vi "Create UI Pointers.vi"(8 "error in (no error)":errorcluster) -> (0 "error out":errorcluster, 3 "UI Pointers":T1)   [LabVIEW 2017]
uses:
  User Interface Pointers.ctl
  <vilib>/NI/Memory Manager/Classes/Pointer/Pointer.lvclass
  <vilib>/NI/Memory Manager/Classes/Pointer/Pointer.lvclass/Pointer.ctl
  <vilib>/NI/Memory Manager/Classes/Pointer/Write U32.vi
  <vilib>/NI/Memory Manager/Classes/Pointer/Write Bool.vi
  <vilib>/NI/Memory Manager/Classes/Pointer/Set Address.vi
  <vilib>/NI/Memory Manager/Classes/Pointer/Set Size.vi
  <vilib>/NI/Memory Manager/Classes/Pointer/Set Internal.vi
  <vilib>/NI/Memory Manager/Classes/Pointer/Clear.vi
  <vilib>/NI/Memory Manager/Classes/Pointer/Write (No Check).vi
  <vilib>/NI/Memory Manager/Classes/Pointer/Write (No Check) U32.vi
  <vilib>/NI/Memory Manager/Classes/Pointer/Check Move.vi
  <vilib>/NI/Memory Manager/Classes/Pointer/Write (No Check) Bool.vi
  <vilib>/NI/Memory Manager/Classes/Pointer/Check Null Pointer.vi
  <vilib>/NI/Memory Manager/Classes/Pointer/Clear (No Check).vi
  <vilib>/NI/Memory Manager/Classes/Pointer/Check Length.vi
  <vilib>/NI/Memory Manager/Classes/Pointer/Get Address.vi
  <vilib>/NI/Memory Manager/Classes/Pointer/Check Count.vi
  <vilib>/NI/Memory Manager/Classes/Pointer/Check Bounds (Power of 2).vi
  <vilib>/NI/Memory Manager/Classes/Pointer/Errors.vi
  <vilib>/NI/Memory Manager/Classes/Pointer/Null Pointer.vi
  <vilib>/NI/Memory Manager/Classes/Pointer/Is Null.vi
  <vilib>/NI/Memory Manager/Classes/Pointer/Get Size.vi
  <vilib>/NI/Memory Manager/Classes/Pointer/Check Bounds (Pointer).vi
  <vilib>/NI/Memory Manager/Classes/Pointer/Out of Bounds.vi
  <vilib>/NI/Memory Manager/Classes/Pointer/Check Bounds.vi
  <vilib>/NI/Memory Manager/Classes/Pointer/Create Error.vi
  <vilib>/NI/Memory Manager/Classes/Pointer/Write Pointer Size to Error.vi
  <vilib>/NI/Memory Manager/Classes/Pointer/Check Bounds (Buffer).vi
  <vilib>/NI/Memory Manager/Constants/Constants.vi
  <vilib>/NI/Memory Manager/Constants/Library Name.vi
  <vilib>/NI/Memory Manager/Classes/Pointer/Pointer Error Info.vi
  <vilib>/NI/Memory Manager/Constants/Pointer Class Name.vi
  <vilib>/NI/Memory Manager/Classes/Pointer/Buffer Underflow.vi
  <vilib>/NI/Memory Manager/VIs/New Error Cluster.vi
  <vilib>/NI/Memory Manager/VIs/New Error Cluster (512B).vi
  <vilib>/NI/Memory Manager/VIs/Set Error Status.vi
  <vilib>/NI/Memory Manager/VIs/Set Error Code.vi
  <vilib>/NI/Memory Manager/VIs/Set Error Source.vi
  <vilib>/NI/Memory Manager/VIs/Write String to Source.vi
  <vilib>/NI/Memory Manager/VIs/Write Numeric to Source.vi
  <vilib>/NI/Memory Manager/VIs/Write Numeric Scalar to Source (Base10 U64).vi
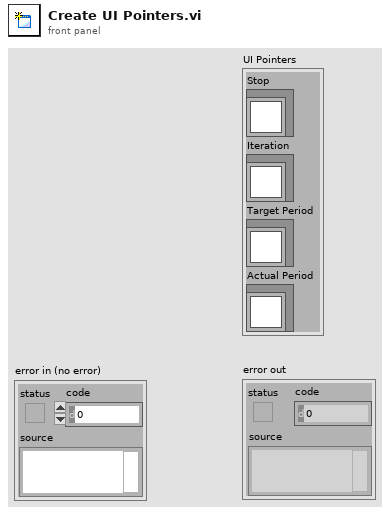
[diagram p1: front panel]
types:
  T1 = typedef "User Interface Pointers.ctl" = cluster{"Stop":refnum<class "Pointer.lvclass">, "Iteration":refnum<class "Pointer.lvclass">, "Target Period":refnum<class "Pointer.lvclass">, "Actual Period":refnum<class "Pointer.lvclass">}
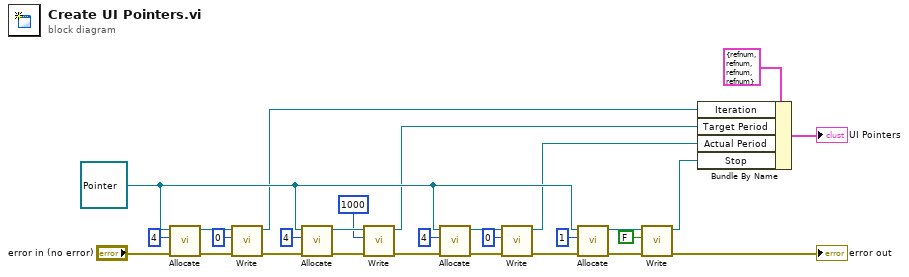
[diagram p0: block diagram]
diagram:
  w13 = refnum<class "Pointer.lvclass"> refnum ("Pointer in")
  n1 = call <vilib>:"Allocate.vi"("error in (no error)"="error in (no error)", "size"=u64 4, "Pointer type"=w13) -> ("error out"=w18:errorcluster, "Pointer out"=w19:refnum<class "Pointer.lvclass">)  [unwired: 7 in]
  n2 = call-poly <vilib>:"Write.vi"("error in (no error)"=w18, "value"=u32 0, "Pointer in"=w19) -> ("error out"=w17:errorcluster, "Pointer out"=w1:refnum<class "Pointer.lvclass">)  [unwired: 5 in, 2 out]
  n3 = call <vilib>:"Allocate.vi"("error in (no error)"=w17, "size"=u64 4, "Pointer type"=w13) -> ("error out"=w23:errorcluster, "Pointer out"=w24:refnum<class "Pointer.lvclass">)  [unwired: 7 in]
  n4 = call-poly <vilib>:"Write.vi"("error in (no error)"=w23, "value"=u32 1000, "Pointer in"=w24) -> ("error out"=w22:errorcluster, "Pointer out"=w2:refnum<class "Pointer.lvclass">)  [unwired: 5 in, 2 out]
  n5 = call <vilib>:"Allocate.vi"("error in (no error)"=w22, "size"=u64 4, "Pointer type"=w13) -> ("error out"=w21:errorcluster, "Pointer out"=w25:refnum<class "Pointer.lvclass">)  [unwired: 7 in]
  n6 = call-poly <vilib>:"Write.vi"("error in (no error)"=w21, "value"=u32 0, "Pointer in"=w25) -> ("error out"=w20:errorcluster, "Pointer out"=w3:refnum<class "Pointer.lvclass">)  [unwired: 5 in, 2 out]
  n7 = call <vilib>:"Allocate.vi"("error in (no error)"=w20, "size"=u64 1, "Pointer type"=w13) -> ("error out"=w28:errorcluster, "Pointer out"=w27:refnum<class "Pointer.lvclass">)  [unwired: 7 in]
  n8 = call-poly <vilib>:"Write.vi"("error in (no error)"=w28, "value"=FALSE, "Pointer in"=w27) -> ("error out"=→"error out":errorcluster, "Pointer out"=w4:refnum<class "Pointer.lvclass">)  [unwired: 5 in, 2 out]
  n9 = Bundle By Name(cluster=T1 {"Stop"=refnum, "Iteration"=refnum, "Target Period"=refnum, "Actual Period"=refnum} ("UI Pointers"), "Iteration"=w1, "Target Period"=w2, "Actual Period"=w3, "Stop"=w4) -> (→"UI Pointers":T1)
